vi "Reset.vi"() -> ()   [LabVIEW 2018]
uses:
  <vilib>/Plasmionique/MB Master/MB_Master_TCP/MB_Master_TCP.lvclass
  C:/Program Files (x86)/National Instruments/LabVIEW 2018/vi.lib/Plasmionique/MB Master/MB_Master/MB_Master.lvclass
  <vilib>/Plasmionique/MB Master/MB Master.lvlib
panel:
  in  "IP Address":string="localhost"
  in  "Stop Button":bool
  in  "Reset":bool
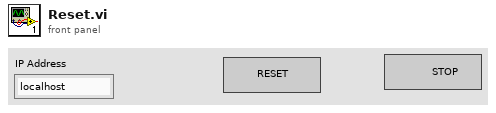
[diagram p1: front panel]
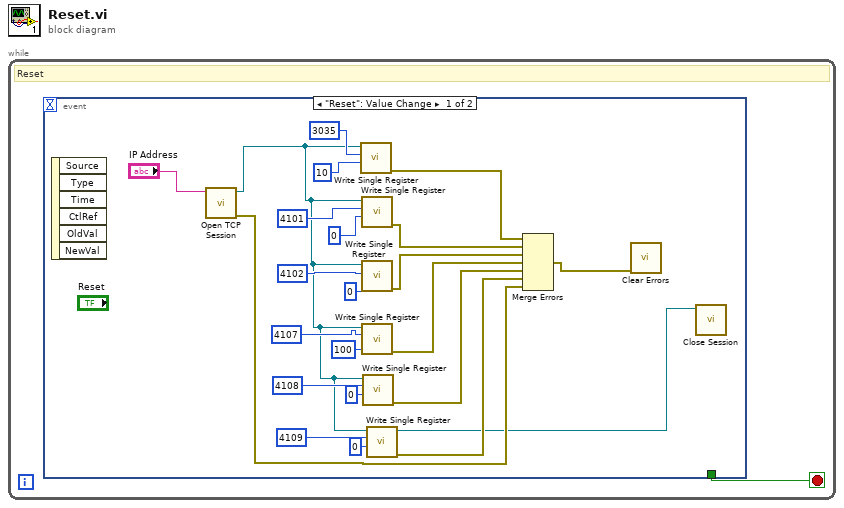
[diagram p0: block diagram]
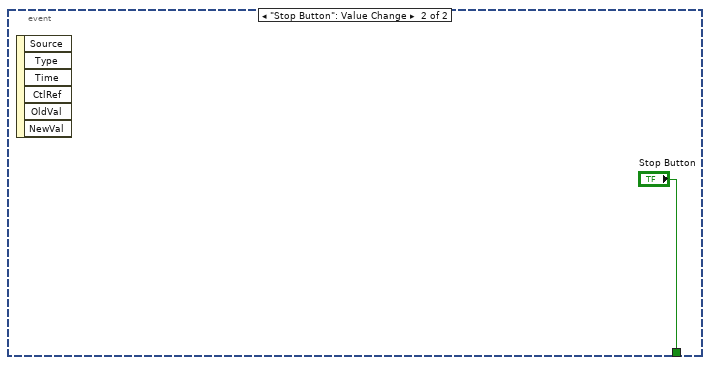
[diagram p2: hidden frame]
diagram:
  n1 = while {
    stop <- w1 stop-if-true
    # "Reset"
    n2 = event shown="[0] \"Reset\": Value Change" {
      selector: _ -> [_ _]
      dyn-events: _ -> [_ _]
      timeout: _ -> [_ _]
      tunnel: [_ "Stop Button"] -> w1
      event "Reset": Value Change {
        n3 = event-data() -> ()  [unwired: 1 in, 6 out]
        n4 = call <vilib>:"Open TCP Session.vi"("IP Address"="IP Address") -> ("error out"=w3:errorcluster, "MB_TCP session"=w11:refnum<class "MB_Master_TCP.lvclass">)  [unwired: 9 in]
        n5 = call <vilib>:"Write Single Register.vi"("value"=u16 10, "address"=u16 3035, "MB session in"=w11) -> ("error out"=w10:errorcluster)  [unwired: 7 in, 1 out]
        n6 = call <vilib>:"Write Single Register.vi"("value"=u16 0, "address"=u16 4101, "MB session in"=w11) -> ("error out"=w9:errorcluster)  [unwired: 7 in, 1 out]
        n7 = call <vilib>:"Write Single Register.vi"("value"=u16 0, "address"=u16 4102, "MB session in"=w11) -> ("error out"=w8:errorcluster)  [unwired: 7 in, 1 out]
        n8 = call <vilib>:"Write Single Register.vi"("value"=u16 100, "address"=u16 4107, "MB session in"=w11) -> ("error out"=w7:errorcluster)  [unwired: 7 in, 1 out]
        n9 = call <vilib>:"Write Single Register.vi"("value"=u16 0, "address"=u16 4108, "MB session in"=w11) -> ("error out"=w6:errorcluster)  [unwired: 7 in, 1 out]
        n10 = call <vilib>:"Write Single Register.vi"("value"=u16 0, "address"=u16 4109, "MB session in"=w11) -> ("error out"=w5:errorcluster, "MB session out"=w2:refnum<class "MB_Master_TCP.lvclass">)  [unwired: 7 in]
        n11 = Merge Errors(w10, w9, w8, w7, w6, w5, w3) -> (w4:errorcluster)
        n12 = call <vilib>:"Clear Errors.vi"("error in (no error)"=w4) -> ()  [unwired: 5 in, 2 out]
        n13 = call-dynamic "Close Session.vi"("MB TCP session"=w2) -> ()  [unwired: 10 in, 1 out]
      }
      event "Stop Button": Value Change {
        n14 = event-data() -> ()  [unwired: 1 in, 6 out]
      }
    }
  }
